vi "GetTerms3.vi"(0 "XRef":T10, 1 "State In":T9={"Input Type"=variant(path path ""), "Terminals"=[]}) -> (14 "Terms":T1)   [LabVIEW 2015, in "Await.xnode"]
doc: "This ability VI is used to describe your terminals to LabVIEW. Terms is an array of clusters describing the XNode's terminals.\n ID: A unique string identifying the terminal.\n Name: The name of the terminal visible to the user. Remember to localize it.\n Type: The data type of the terminal (as a Variant). The data put in the variant will be used as the default for the input terminal if it's left unwired.\n Bounds: A rectangle defining the bounds of the terminal relative to the bounds of the XNode. The bounds must be within the bounds of the XNode, and for whiskers to draw properly, they must be flush with at least one side of the XNode.\n Input?: Indicates whether or not this terminals is an input.\n Required?: Indicates whether the user must wire this terminal for the XNode to not be broken. Ignored on outputs.\n Recommended?: Indicates whether the terminal is recommended.\n Hidden?: Indicates whether the terminal is hidden. When a terminal is hidden, it cannot be wired to via user interaction or scripting. However, if it is already wired to when the hidden flag is changed to true, it will remain wired.\n Adaptive?: Indicates that the term should change to match the type of its source if it is wired.\n Direction?: Indicates what direction the wire stub should point. Choose auto to let LV decide based on the terms bounds being on the nodes edge.\n \n The IDs are used by LabVIEW to keep track of your terminals. When you respecify your terminals, LabVIEW can tell whther terminals are new, deleted, or moved by the unique IDs. The order is irrelevant. If you move a terminal, then any wire connected to it will move with it.\n \n If you want to update your terminals, you should return the UpdateTerms reply in one of your ability VIs.\n\nDefault behavior: None.\n\nThis ability does not provide UI and OS messages are not handled."
uses:
  Await.xnode
  <vilib>/XNodeSupport/XNodeXNodeRef.ctl
  State.ctl
  <vilib>/XNodeSupport/XNodeTerm3Array.ctl
  <vilib>/XNodeSupport/XNodeTerm3.ctl
  <vilib>/XNodeSupport/XNodeString.ctl
  <vilib>/XNodeSupport/XNodeVariant.ctl
  <vilib>/XNodeSupport/XNodeRect32.ctl
  <vilib>/XNodeSupport/XNodeInt.ctl
  <vilib>/XNodeSupport/XNodeBool.ctl
  <vilib>/XNodeSupport/XNodeTermDirection.ctl
  <vilib>/Utility/miscctls.llb/LVRectTypeDef.ctl
  <vilib>/Utility/Data Type/Type Definitions/Data Type.ctl
  <vilib>/XNodeSupport/NI_XNodeSupport.lvlib
  <vilib>/Utility/Data Type/NI_Data Type.lvlib
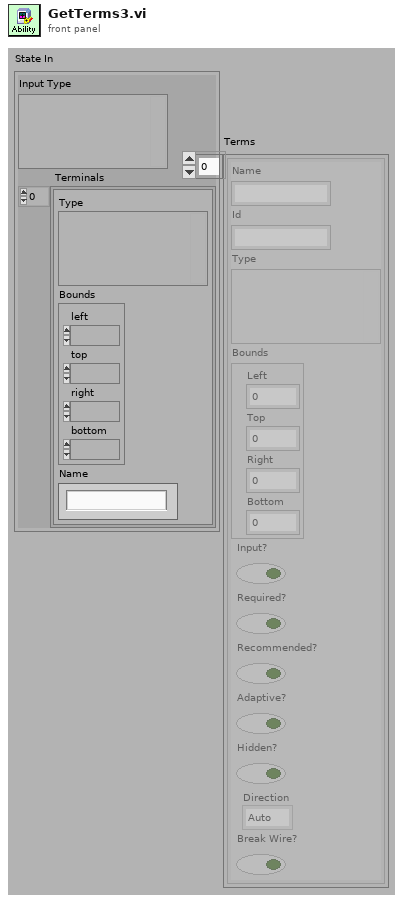
[diagram p1: front panel]
types:
  T1 = typedef "NI_XNodeSupport.lvlib/XNodeTerm3Array.ctl" = T2[]
  T2 = typedef "NI_XNodeSupport.lvlib/XNodeTerm3.ctl" = cluster{"Name":T3, "Id":T3, "Type":T4, "Bounds":T5, "Input?":T7, "Required?":T7, "Recommended?":T7, "Adaptive?":T7, "Hidden?":T7, "Direction":T8, "Break Wire?":T7}
  T3 = typedef "NI_XNodeSupport.lvlib/XNodeString.ctl" = string
  T4 = typedef "NI_XNodeSupport.lvlib/XNodeVariant.ctl" = variant
  T5 = typedef "NI_XNodeSupport.lvlib/XNodeRect32.ctl" = cluster{"Left":T6, "Top":T6, "Right":T6, "Bottom":T6}
  T6 = typedef "NI_XNodeSupport.lvlib/XNodeInt.ctl" = i32
  T7 = typedef "NI_XNodeSupport.lvlib/XNodeBool.ctl" = bool
  T8 = typedef "NI_XNodeSupport.lvlib/XNodeTermDirection.ctl" = enum32{"Auto", "Up", "Down", "Left", "Right", "Center"}
  T9 = typedef "Await.xnode/State.ctl" = cluster{"Input Type":variant, "Terminals":cluster{"Type":variant, "Bounds":cluster{"left":i16, "top":i16, "right":i16, "bottom":i16}, "Name":string}[]}
  T10 = typedef "NI_XNodeSupport.lvlib/XNodeXNodeRef.ctl" = refnum<vi>
  T11 = cluster{"Type":variant, "Bounds":cluster{"left":i16, "top":i16, "right":i16, "bottom":i16}, "Name":string}[]
  T12 = typedef "LVRectTypeDef.ctl" = cluster{"Left":i16, "Top":i16, "Right":i16, "Bottom":i16}
  T13 = typedef "NI_Data Type.lvlib/Data Type.ctl" = enum8{"Invalid Type", "Void", "I8", "I16", "I32", "I64", "U8", "U16", "U32", "U64", "Single Float", "Double Float", "Extended Float", "Single Complex", "Double Complex", "Extended Complex", "Enum U8", "Enum U16", "Enum U32", "Enum U64", "Single Float With Unit", "Double Float With Unit", "Extended Float With Unit", "Single Complex with Unit", "Double Complex with Unit", "Extended Complex with Unit", "Boolean", "String", "Path", "Picture", "Tag", "Array", "Cluster", "Variant", "LV Variant", "Waveform", "Timestamp", "Digital Waveform", "Digital Data", "ExpressData", "Refnum", "External Data", "VI", "Poly VI", "LabVIEW Class Instance", "Fixed Point"}
  T14 = cluster{"left":i16, "top":i16, "right":i16, "bottom":i16}
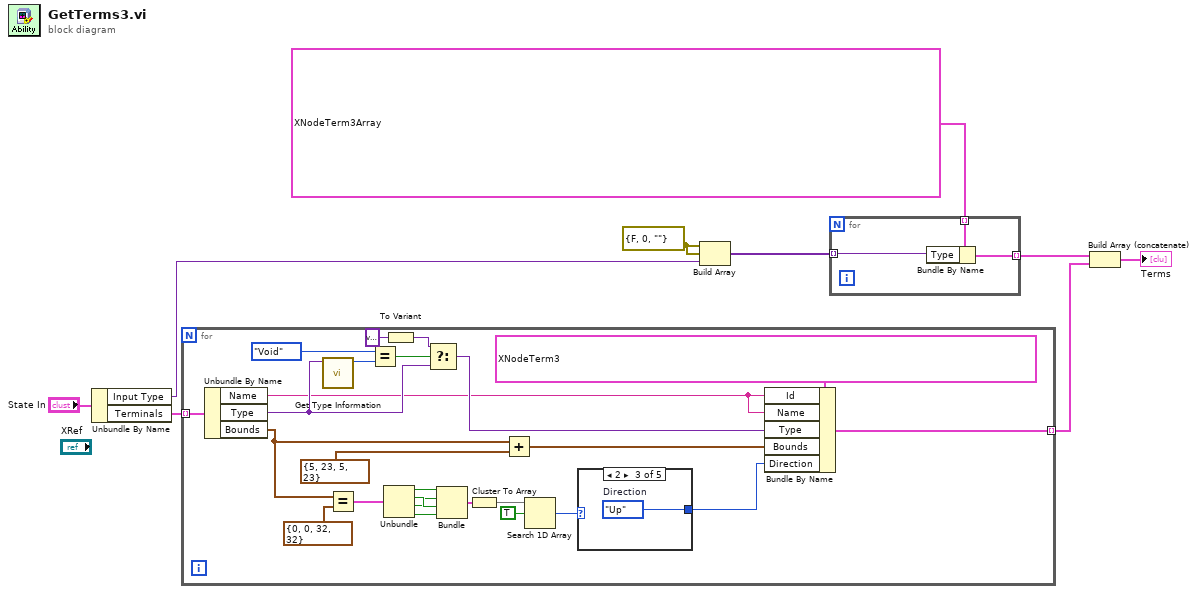
[diagram p0: block diagram]
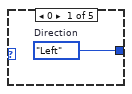
[diagram p2: hidden frame]
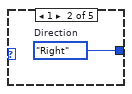
[diagram p3: hidden frame]
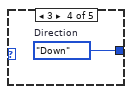
[diagram p4: hidden frame]
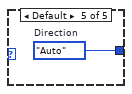
[diagram p5: hidden frame]
diagram:
  w2 = errorcluster {"status"=FALSE, "code"=0, "source"=""} ("error constant")
  n1 = Unbundle By Name("State In") -> ("Input Type"=w1:variant, "Terminals"=w8:T11)
  n2 = for {
    tunnel: w8 -> [w34] mode=indexing
    tunnel: [w31] -> w5 mode=indexing
    n3 = Unbundle By Name(w34) -> ("Name"=w11:string, "Type"=w18:variant, "Bounds"=w22:T14)
    n4 = call <vilib>:"Get Type Information.vi"("Variant"=w18) -> ("Type"=w28:T13)  [unwired: 6 in, 4 out]
    n5 = Equal?(x=w22, y=T12 {"Left"=0, "Top"=0, "Right"=32, "Bottom"=32}) -> (x = y?=w17:cluster{bool, bool, bool, bool})
    n6 = Equal?(x=Data_Type."Void", y=w28) -> (x = y?=w26:bool)
    n7 = Unbundle(w17) -> (w16:bool, w15:bool, w14:bool, w13:bool)
    n8 = To Variant(anything=variant) -> (Variant=w25:variant)
    n9 = Select(t=w25, s=w26, f=w18) -> (s? t:f=w24:variant)
    n10 = Bundle(w16, w14, w15, w13) -> (w12:cluster{bool, bool, bool, bool})  [unwired: 1 in]
    n11 = Cluster To Array(cluster=w12) -> (array=w33:bool[])
    n12 = Add(x=w22, y=T12 {"Left"=5, "Top"=23, "Right"=5, "Bottom"=23}) -> (x+y=w30:T12)
    n13 = Search 1D Array(1D array=w33, element=TRUE) -> (index of element=w32:i32)  [unwired: 1 in]
    n14 = case shown="2" w32 {
      tunnel: [w35 w36 w37 w38 w39] -> w19
      frame 0 {
        w35 = XNodeTermDirection."Left"  # Direction
      }
      frame 1 {
        w36 = XNodeTermDirection."Right"  # Direction
      }
      frame 2 {
        w37 = XNodeTermDirection."Up"  # Direction
      }
      frame 3 {
        w38 = XNodeTermDirection."Down"  # Direction
      }
      frame Default {
        w39 = XNodeTermDirection."Auto"  # Direction
      }
    }
    n15 = Bundle By Name(cluster=T2 {"Name"="", "Id"="", "Type"=variant, "Bounds"={"Left"=0, "Top"=0, "Right"=0, "Bottom"=0}, "Input?"=FALSE, "Required?"=FALSE, "Recommended?"=FALSE, "Adaptive?"=FALSE, "Hidden?"=FALSE, "Direction"=enum."Auto", "Break Wire?"=FALSE} ("Term 3"), "Id"=w11, "Name"=w11, "Type"=w24, "Bounds"=w30, "Direction"=w19) -> (w31:T2)
  }
  n16 = Build Array(w2, w2, w1) -> (w3:variant[])
  n17 = for {
    tunnel: T1 [{"Name"="Error In", "Id"="ein", "Type"=variant, "Bounds"={"Left"=0, "Top"=9, "Right"=8, "Bottom"=17}, "Input?"=TRUE, "Required?"=FALSE, "Recommended?"=FALSE, "Adaptive?"=FALSE, "Hidden?"=FALSE, "Direction"=enum."Auto", "Break Wire?"=FALSE}, {"Name"="Error Out", "Id"="eout", "Type"=variant, "Bounds"={"Left"=34, "Top"=9, "Right"=42, "Bottom"=17}, "Input?"=FALSE, "Required?"=FALSE, "Recommended?"=FALSE, "Adaptive?"=FALSE, "Hidden?"=FALSE, "Direction"=enum."Auto", "Break Wire?"=FALSE}, {"Name"="VI Ref", "Id"="viref", "Type"=variant, "Bounds"={"Left"=0, "Top"=1, "Right"=8, "Bottom"=8}, "Input?"=TRUE, "Required?"=TRUE, "Recommended?"=FALSE, "Adaptive?"=FALSE, "Hidden?"=FALSE, "Direction"=enum."Left", "Break Wire?"=FALSE}] ("Terms") -> [w42] mode=indexing
    tunnel: [w41] -> w6 mode=indexing
    tunnel: w3 -> [w40] mode=indexing
    n18 = Bundle By Name(cluster=w42, "Type"=w40) -> (w41:T2)
  }
  n19 = Build Array (concatenate)(w6, w5) -> (→"Terms":T2[])
